vi "CHECKSN.vi"(9 "SN":string, 10 "menu reference":refnum<k9>) -> (1 "SNCheck":bool)   [LabVIEW 2013]
uses:
  Control/Buffer.vi
panel:
  in  "CheckInmsFlow._CheckFlow":refnum<k7>
  out "CheckInmsFlow":i16
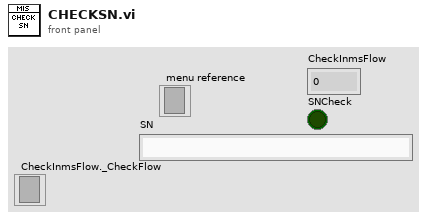
[diagram p1: front panel]
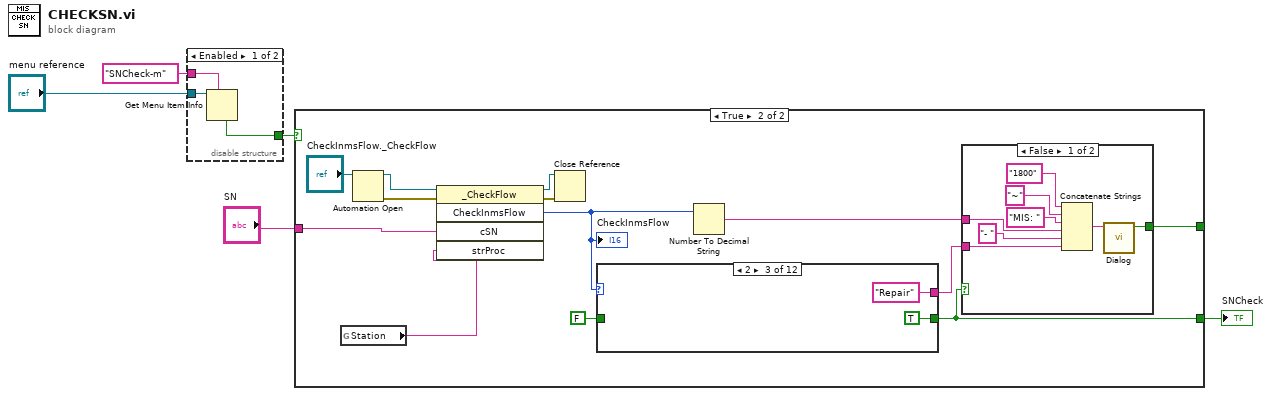
[diagram p0: block diagram]
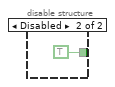
[diagram p2: hidden frame]
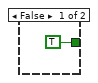
[diagram p3: hidden frame]
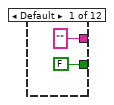
[diagram p5: hidden frame]
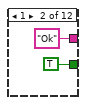
[diagram p6: hidden frame]
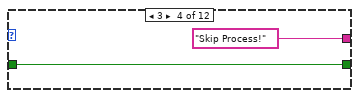
[diagram p7: hidden frame]
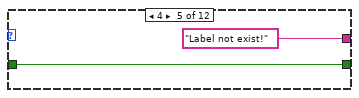
[diagram p8: hidden frame]
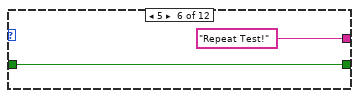
[diagram p9: hidden frame]
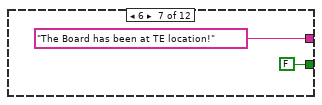
[diagram p10: hidden frame]
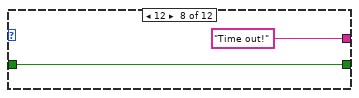
[diagram p11: hidden frame]
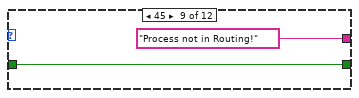
[diagram p12: hidden frame]
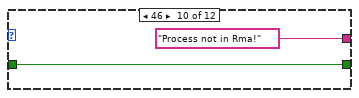
[diagram p13: hidden frame]
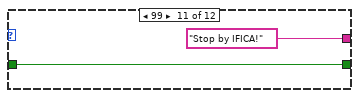
[diagram p14: hidden frame]
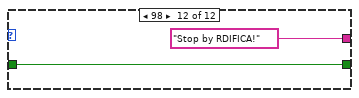
[diagram p15: hidden frame]
diagram:
  n1 = disable-structure shown="Enabled" {
    disable-tunnel: "menu reference" -> [w8 _]
    disable-tunnel: "SNCheck-m" ("item tag") -> [w7 _]
    disable-tunnel: [w6 TRUE ("checked")] -> w4
    frame Enabled {
      n2 = Get Menu Item Info(7:w7, 11:w8) -> (4:w6:bool)  [unwired: 1 in, 6 out]
    }
    frame Disabled {
    }
  }
  n3 = case shown="True" w4 {
    tunnel: [TRUE w14] -> w3
    tunnel: [_ w19] -> _
    tunnel: "SN" -> [_ w13]
    frame False {
    }
    frame True {
      n4 = global read "Buffer.vi" "Station"() -> (w12:string)
      n5 = Automation Open(Automation Refnum="CheckInmsFlow._CheckFlow") -> (Automation Refnum=w23:refnum<k7>, error out=w21:errorcluster)  [unwired: 3 in]
      n6 = invoke class="_CheckFlow" method="CheckInmsFlow"(reference=w23, error in=w21, "cSN"=w13, "strProc"=w12) -> (reference out=w22:refnum<k7>, error out=w20:errorcluster, "CheckInmsFlow"=w16:i16)  [unwired: 1 in, 2 out]
      "CheckInmsFlow" <- w16
      n7 = Close Reference(reference=w22, error in (no error)=w20) -> ()  [unwired: 1 out]
      n8 = case shown="2" w16 {
        tunnel: [FALSE TRUE TRUE w39 w41 w43 FALSE w47 w49 w51 w53 w55] -> w14
        tunnel: ["" "Ok" "Repair" "Skip Process!" "Label not exist!" "Repeat Test!" "The Board has been at TE location!" "Time out!" "Process not in Routing!" "Process not in Rma!" "Stop by IFICA!" "Stop by RDIFICA!"] -> w15
        tunnel: FALSE -> [_ _ _ w39 w41 w43 _ w47 w49 w51 w53 w55]
        frame Default {
        }
        frame 1 {
        }
        frame 2 {
        }
        frame 3 {
        }
        frame 4 {
        }
        frame 5 {
        }
        frame 6 {
        }
        frame 12 {
        }
        frame 45 {
        }
        frame 46 {
        }
        frame 99 {
        }
        frame 98 {
        }
      }
      n9 = Number To Decimal String(number=w16) -> (decimal integer string=w17:string)  [unwired: 1 in]
      n10 = case shown="False" w14 {
        tunnel: [w27 _] -> w19
        tunnel: w17 -> [w26 _]
        tunnel: w15 -> [w24 _]
        frame False {
          n11 = Concatenate Strings("1800" ("string"), "~" ("string"), "MIS: ", w26, "- " ("string"), w24) -> (w30:string)
          n12 = call "Dialog.vi"("Limit"=w30) -> ("true"=w27:bool)  [unwired: 9 in, 1 out]
        }
        frame True {
        }
      }
    }
  }
  "SNCheck" <- w3
